vi "AverageArray.vi"(1 "Input Array":dbl[](array[numeric]), 2 "Samples To Average":i32) -> (0 "Averaged Array":dbl[](array[numeric]))   [LabVIEW 2012]
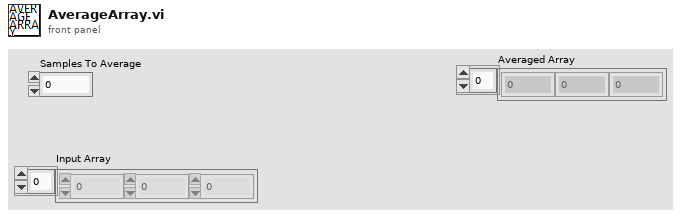
[diagram p1: front panel]
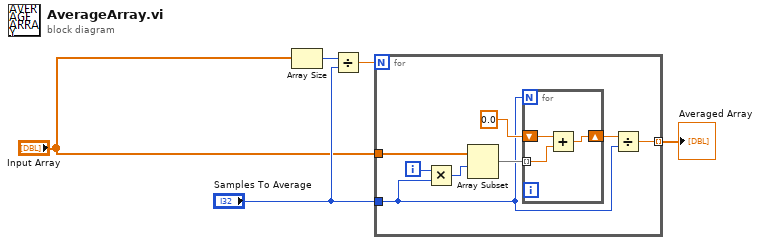
[diagram p0: block diagram]
diagram:
  n1 = Array Size(array="Input Array") -> (size(s)=w4:i32)
  n2 = Divide(x=w4, y="Samples To Average") -> (x/y=w2:dbl)
  n3 = for {
    N: w2 -> [_]
    tunnel: "Samples To Average" -> [w7]
    tunnel: [w6] -> w5 mode=indexing
    tunnel: "Input Array" -> [w9]
    i -> [w12]
    n4 = Multiply(x=w12, y=w7) -> (x*y=w10:i32)
    n5 = Array Subset(array=w9, index=w10) -> (w11:dbl[])  [unwired: 1 in]
    n6 = for {
      N: w7 -> [_]
      tunnel: w11 -> [w14] mode=indexing
      shift-right: [w16] -> w8
      shift-left: 0.0 -> [w15]
      n7 = Add(x=w15, y=w14) -> (x+y=w16:dbl)
    }
    n8 = Divide(x=w8, y=w7) -> (x/y=w6:dbl)
  }
  "Averaged Array" <- w5
